vi "Agilent 34970 RF Mux.vi"() -> ()   [LabVIEW 2016]
doc: "This VI shows you how to use the 34905A RF Mux. For each of the two multiplexers, specify the channel you wish to close . Each multiplexer has 4 channels."
uses:
  Agilent 34970.lvlib
panel:
  in  "Serial Port Configuration":T1={"Timeout Value (10000)"=10000, "Baud Rate (57600)"=enum."57600", "Flow Control (1:XON/XOFF)"=enum."XON / XOFF"}
  in  "Reset":bool=TRUE
  in  "VISA resource name":refnum<visa-resource-name>
  in  "Slot Number":u16=1 min=1 max=3 step=1
  in  "Mux 2":u8=1 min=1 max=4 step=1
  in  "Mux 1":u8=1 min=1 max=4 step=1
  # "(c) 2005-2010 National Instruments.  ALL RIGHTS RESERVED."
  # "Channels to Close"
  # "This VI shows how to use the RF multiplexer on the HP34907A module.\n\nThe HP34907A has two banks which have 4 channels each.  Only one chanel may be closed on each bank.\n\nSet the Slot Number control to specify which slot the HP34907A is in."
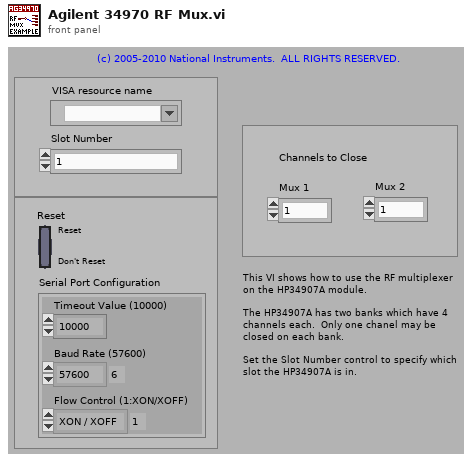
[diagram p1: front panel]
types:
  T1 = cluster{"Timeout Value (10000)":u32, "Baud Rate (57600)":enum16{"1200", "2400", "4800", "9600", "19200", "38400", "57600", "115200"}, "Flow Control (1:XON/XOFF)":enum16{"None", "XON / XOFF", "RTS / CTS", "DTR / DSR"}}
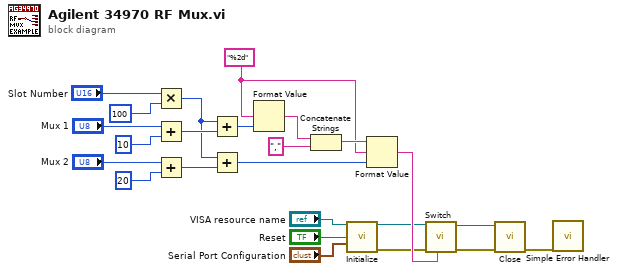
[diagram p0: block diagram]
diagram:
  w9 = "%2d" ("format string")
  n1 = Multiply(x="Slot Number", y=u16 100) -> (x*y=w12:u16)
  n2 = Add(x="Mux 1", y=u8 10) -> (x+y=w18:u8)
  n3 = Add(x="Mux 2", y=u8 20) -> (x+y=w19:u8)
  n4 = Add(x=w12, y=w18) -> (x+y=w14:u16)
  n5 = Add(x=w12, y=w19) -> (x+y=w13:u16)
  n6 = Format Value(format string=w9, value (0)=w14) -> (output string=w17:string)  [unwired: 1 in]
  n7 = Concatenate Strings(w17, ",") -> (w15:string)
  n8 = call "Initialize.vi"("VISA Resource Name"="VISA resource name", "Reset (T: Reset)"="Reset", "Serial Port Configuration"="Serial Port Configuration") -> ("VISA Resource Name Out"=w8:refnum<visa-resource-name>, "error out"=w7:errorcluster)  [unwired: 11 in]
  n9 = Format Value(string ("")=w15, format string=w9, value (0)=w13) -> (output string=w11:string)
  n10 = call "Switch.vi"("Channel List(empty)"=w11, "error in (no error)"=w7, "VISA Resource Name"=w8) -> ("error out"=w5:errorcluster, "VISA Resource Name Out"=w6:refnum<visa-resource-name>)  [unwired: 6 in, 1 out]
  n11 = call "Close.vi"("VISA Resource Name"=w6, "error in (no error)"=w5) -> ("error out"=w1:errorcluster)  [unwired: 13 in]
  n12 = call <vilib>:"Simple Error Handler.vi"("error in (no error)"=w1) -> ()  [unwired: 4 in, 5 out]
